vi "Test Time Measurement.vi"() -> (2 "ICov Testing time (seconds)":dbl, 3 "UTF Testing time (seconds)":dbl)   [LabVIEW 2018]
uses:
  <vilib>/utf/common/utf_test_result.ctl
  <vilib>/addons/_JKI Toolkits/VI Tester/VI Tester API.llb/Run Tests (Path).vi
  <resource>/Framework/Providers/InstaCoverage/Core/TestSuite/Read UserResultEnum.vi
  <vilib>/utf/NI_UnitTestFramework.lvlib
  <resource>/Framework/Providers/InstaCoverage/Pro/InstaCoveragePro.lvlib
  <vilib>/addons/_JKI Toolkits/VI Tester/VI Tester API.llb/VI Tester API.lvlib
  <resource>/Framework/Providers/InstaCoverage/Core/TestSuite/TestSuite.lvclass
panel:
  out "Caraya In Progress":bool
  out "Caraya report":string
  out "VI Tester report":string
  out "Caraya Testing time (seconds)":dbl
  out "VI Tester In Progress":bool
  out "VI Tester Testing time (seconds)":dbl
  out "ICov Results":enum16{"PASSED", "FAILED", "ERROR"}[](array[ring])
  out "ICov In Progress":bool
  out "UTF In Progress":bool
  out "UTF Results":T1[](array[typedef])
  out "Project Path":string
  # "UTF"
  # "ICov"
  # "VI Tester"
  # "Caraya"
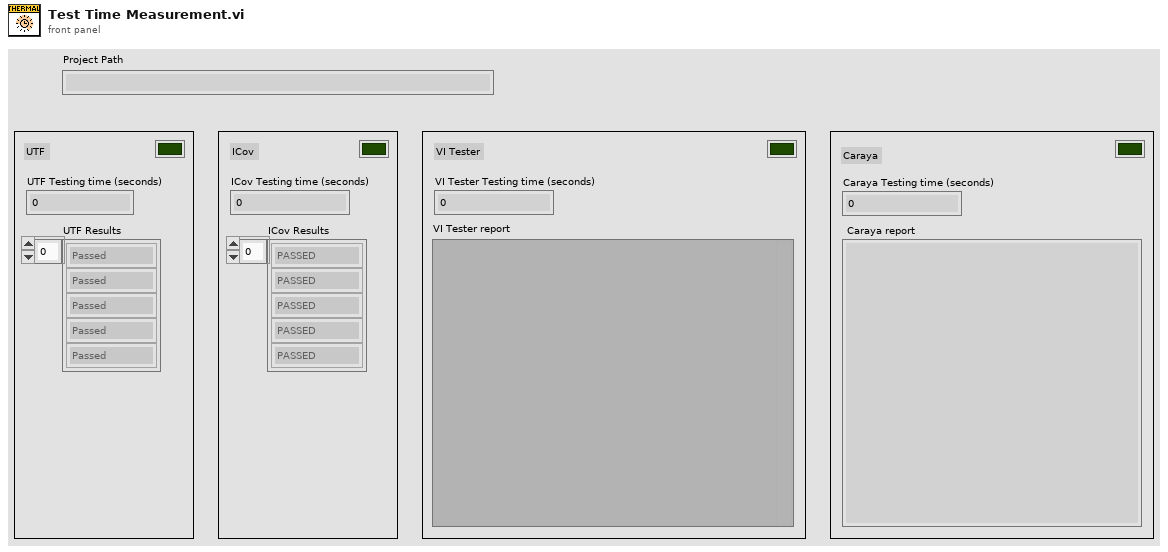
[diagram p1: front panel]
types:
  T1 = typedef "NI_UnitTestFramework.lvlib/utf_test_result.ctl" = enum16{"Passed", "Failed", "Error", "Skipped", "Not Processed"}
  T2 = typedef "NI_UnitTestFramework.lvlib/utf_test_result_overall.ctl" = cluster{"utf results out":T3[], "untested VIs":cluster{"VI path":path, "code coverage":T11, "vi hierarchy":string[]}[], "project file path":path, "system information":string}
  T3 = typedef "NI_UnitTestFramework.lvlib/utf_test_result_testfile.ctl" = cluster{"test case":T4[], "test status":T1, "test path":path, "setup VI":path, "teardown VI":path, "code coverage":T11, "start time":timestamp, "end time":timestamp, "test hierarchy":string[], "VI path":path, "VI timestamp":timestamp, "VI rev hist":i32, "requirements ID":string, "array brackets":string, "name separator":string, "errors":T12[], "paragraph header":string, "result comment":string, "vi hierarchy":string[], "subVI coverage info":T11[], "subVI info":T14[], "big array threshold":u32, "VI Index":i32, "Comment":string, "Dynamic Dispatch":bool, "User-defined test VI":path, "user-defined VI code coverage":T11}
  T4 = typedef "NI_UnitTestFramework.lvlib/utf_test_result_testcase.ctl" = cluster{"test result":T1, "run Times":T5[], "test case name":string, "requirements":string, "code coverage":T11, "subVI coverage info":T11[]}
  T5 = typedef "NI_UnitTestFramework.lvlib/utf_test_result_troll_new.ctl" = cluster{"result (test)":T1, "Vector Result":T6[]}
  T6 = typedef "NI_UnitTestFramework.lvlib/utf_vector_result.ctl" = cluster{"time elapsed [ms]":u32, "result (test)":T1, "result (parameters)":T7[], "Used Vector Values":cluster{"Vector Name":string, "element":i32}[], "Executed Class Path":path, "Input":T10[]}
  T7 = typedef "NI_UnitTestFramework.lvlib/utf_test_result_failure.ctl" = cluster{"result":T1, "error message":string, "parameter name":string, "parameter value":variant, "parameters":variant[], "comparison":T8, "requirement ID":string, "VI":T9, "Used Vector Name":string}
  T8 = typedef "NI_UnitTestFramework.lvlib/utf_test_comparison_operators.ctl" = enum16{"=", "!=", ">", ">=", "<", "<=", "range", "symmetric tolerance", "asymmetric tolerance", "string contains", "string not contain", "array size", "string length", "array range", "by element", "array range (limit array)", "user-defined", "array contains", "array not contain", "vector length", "= (elm)", "!= (elm)", "= (case insensitive)", "!= (case insensitive)"}
  T9 = typedef "NI_UnitTestFramework.lvlib/utf_vi_tag.ctl" = enum16{"Setup VI", "VI under Test", "Teardown VI"}
  T10 = typedef "NI_UnitTestFramework.lvlib/utf_test_result_input_data.ctl" = cluster{"Name":string, "Input Value":variant[], "VI":T9, "Used Vector Index":i32}
  T11 = typedef "NI_UnitTestFramework.lvlib/utf_code_coverage.ctl" = cluster{"coverage":dbl, "diagram run flag":bool[]}
  T12 = typedef "NI_UnitTestFramework.lvlib/utf_error_data.ctl" = cluster{"error type":T13, "description":string}
  T13 = typedef "NI_UnitTestFramework.lvlib/utf_error_type.ctl" = enum16{"TestFileError", "VIError", "SetupVIError", "TearDownVIError", "OtherError"}
  T14 = typedef "NI_UnitTestFramework.lvlib/utf_subvi_info.ctl" = cluster{"Path":path, "Dependence VI":bool}
  T15 = typedef "InstaCoverage.lvlib/InstaCoverageCore.lvlib/UserResultEnum.ctl" = enum16{"PASSED", "FAILED", "ERROR", "NONE", "AVAILABLE IN PRO"}
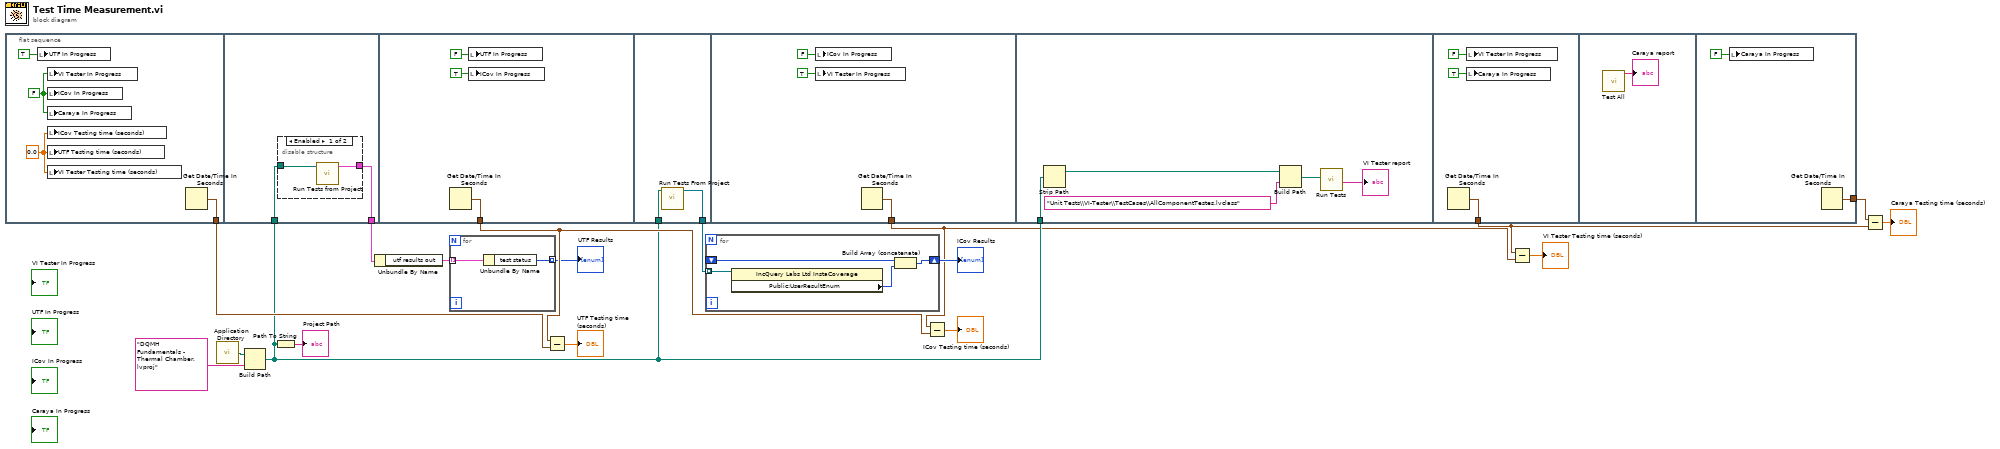
[diagram p0: block diagram]
diagram:
  n1 = flat-sequence {
    tunnel: [w22] -> w13
    tunnel: w6 -> [w24]
    tunnel: [w23] -> w11
    tunnel: [w29] -> w12
    tunnel: w6 -> [w31]
    tunnel: [w30] -> w8
    tunnel: [w34] -> w5
    tunnel: w6 -> [w39]
    tunnel: [w41] -> w1
    tunnel: [w45] -> w2
    frame #0 {
      w19 = FALSE
      w20 = 0.0
      n2 = local write "UTF In Progress"(TRUE) -> ()
      n3 = local write "VI Tester In Progress"(w19) -> ()
      n4 = local write "ICov In Progress"(w19) -> ()
      n5 = local write "Caraya In Progress"(w19) -> ()
      n6 = local write "ICov Testing time (seconds)"(w20) -> ()
      n7 = local write "UTF Testing time (seconds)"(w20) -> ()
      n8 = local write "VI Tester Testing time (seconds)"(w20) -> ()
      n9 = Get Date/Time In Seconds() -> (seconds since 1Jan1904=w22:timestamp)
    }
    frame #1 {
      n10 = disable-structure shown="Enabled" {
        disable-tunnel: w24 -> [w26 _]
        disable-tunnel: [w25 _] -> w23
        frame Enabled {
          n11 = call <resource>:"Run Tests from Project.vi"("project file path"=w26) -> ("test results out"=w25:T2)  [unwired: 9 in, 1 out]
        }
        frame Disabled {
        }
      }
    }
    frame #2 {
      n12 = Get Date/Time In Seconds() -> (seconds since 1Jan1904=w29:timestamp)
      n13 = local write "UTF In Progress"(FALSE) -> ()
      n14 = local write "ICov In Progress"(TRUE) -> ()
    }
    frame #3 {
      n15 = call <resource>:"Run Tests From Project.vi"("Path lvProject"=w31) -> ("TestSuite[] results"=w30:refnum<class "TestSuite.lvclass">[])  [unwired: 9 in, 1 out]
    }
    frame #4 {
      n16 = local write "ICov In Progress"(FALSE) -> ()
      n17 = local write "VI Tester In Progress"(TRUE) -> ()
      n18 = Get Date/Time In Seconds() -> (seconds since 1Jan1904=w34:timestamp)
    }
    frame #5 {
      n19 = Strip Path(path=w39) -> (stripped path=w38:path)  [unwired: 1 out]
      n20 = Build Path(base path=w38, name or relative path="Unit Tests\\VI-Tester\\TestCases\\AllComponentTestes.lvclass") -> (appended path=w36:path)
      n21 = call-poly <vilib>:"Run Tests.vi"("Test Path"=w36) -> ("test details"=→"VI Tester report":string)  [unwired: 8 in, 2 out]
    }
    frame #6 {
      n22 = Get Date/Time In Seconds() -> (seconds since 1Jan1904=w41:timestamp)
      n23 = local write "VI Tester In Progress"(FALSE ("ICov In Progress")) -> ()
      n24 = local write "Caraya In Progress"(TRUE ("ICov In Progress")) -> ()
    }
    frame #7 {
      n25 = call "Test All.vi"() -> ("report"=→"Caraya report":string)  [unwired: 10 in, 1 out]
    }
    frame #8 {
      n26 = local write "Caraya In Progress"(FALSE ("ICov In Progress")) -> ()
      n27 = Get Date/Time In Seconds() -> (seconds since 1Jan1904=w45:timestamp)
    }
  }
  n28 = call <vilib>:"Application Directory.vi"() -> ("Application Directory"=w18:path)
  n29 = Build Path(base path=w18, name or relative path="DQMH Fundamentals - Thermal Chamber.lvproj") -> (appended path=w6:path)
  n30 = Path To String(path=w6) -> (string=→"Project Path":string)
  n31 = Unbundle By Name(w11) -> ("utf results out"=w10:T3[])
  n32 = for {
    tunnel: w10 -> [w47] mode=indexing
    tunnel: [w46] -> w9 mode=indexing
    n33 = Unbundle By Name(w47) -> ("test status"=w46:T1)
  }
  "UTF Results" <- w9
  n34 = Subtract(x=w12, y=w13) -> (x-y=→"UTF Testing time (seconds)":dbl)
  n35 = for {
    tunnel: w8 -> [w51] mode=indexing
    shift-right: [w48] -> w7
    shift-left: _ -> [w49]
    n36 = property class="IncQuery Labs Ltd InstaCoverage"(reference=w51) -> ("Public:UserResultEnum"=w50:T15)  [unwired: 1 in, 2 out]
    n37 = Build Array (concatenate)(w49, w50) -> (w48:T15[])
  }
  "ICov Results" <- w7
  n38 = Subtract(x=w5, y=w12) -> (x-y=→"ICov Testing time (seconds)":dbl)
  n39 = Subtract(x=w1, y=w5) -> (x-y=→"VI Tester Testing time (seconds)":dbl)
  n40 = Subtract(x=w2, y=w1) -> (x-y=→"Caraya Testing time (seconds)":dbl)
